vi "Execute All Tests.vi"(8 "error in (no error)":errorcluster, 11 "Test Manager in":refnum<class "Test Manager.lvclass">) -> (0 "error out":errorcluster, 3 "Test Manager out":refnum<class "Test Manager.lvclass">)   [LabVIEW 2020, in "Test Manager.lvlib" / "Test Manager.lvclass"]
uses:
  Test Manager.lvclass
  Test Manager.lvclass/Test Manager.ctl
  _Abstract Classes/Test/Test.lvclass
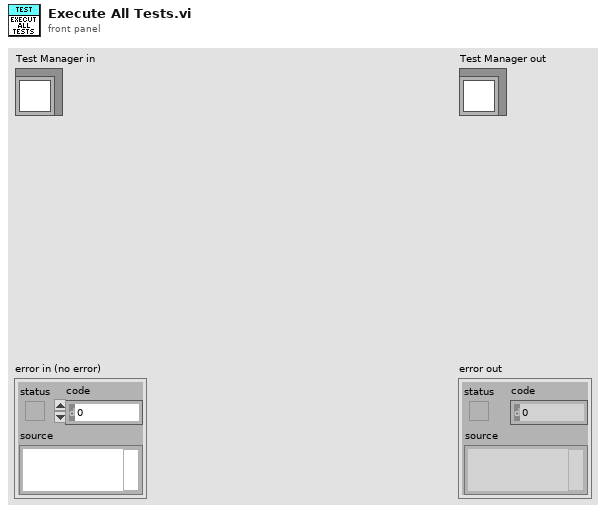
[diagram p1: front panel]
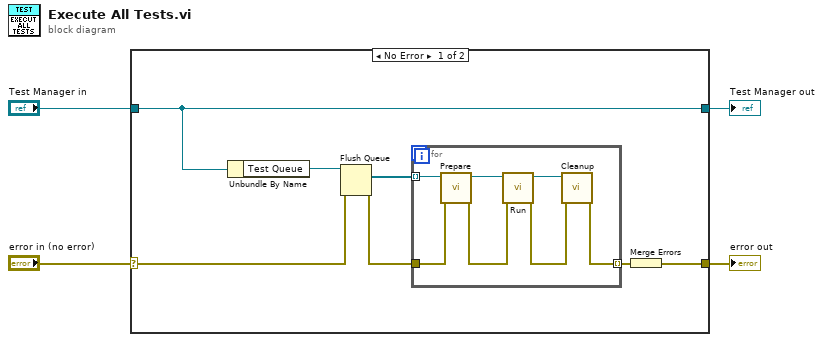
[diagram p0: block diagram]
diagram:
  n1 = case shown="No Error" "error in (no error)" {
    selector: "error in (no error)" -> [w8 w20]
    tunnel: [w5 w20] -> w3
    tunnel: [w11 w19] -> w1
    tunnel: "Test Manager in" -> [w11 w19]
    frame No Error {
      n2 = Unbundle By Name(w11) -> ("Test Queue"=w10:refnum<queue>)
      n3 = Flush Queue(queue=w10, error in (no error)=w8) -> (remaining elements=w9:refnum<class "Test.lvclass">[], error out=w7:errorcluster)  [unwired: 1 out]
      n4 = for {
        tunnel: w9 -> [w14] mode=indexing
        tunnel: w7 -> [w13]
        tunnel: [w12] -> w6 mode=indexing
        n5 = call-dynamic "Prepare.vi"("error in (no error)"=w13, "Test in"=w14) -> ("error out"=w16:errorcluster, "Test out"=w18:refnum<class "Test.lvclass">)  [unwired: 8 in]
        n6 = call-dynamic "Run.vi"("error in (no error)"=w16, "Test in"=w18) -> ("error out"=w15:errorcluster, "Test out"=w17:refnum<class "Test.lvclass">)  [unwired: 8 in]
        n7 = call-dynamic "Cleanup.vi"("error in (no error)"=w15, "Test in"=w17) -> ("error out"=w12:errorcluster)  [unwired: 8 in, 1 out]
      }
      n8 = Merge Errors(w6) -> (w5:errorcluster)
    }
    frame Error {
    }
  }
  "error out" <- w3
  "Test Manager out" <- w1
